vi "Get Configuration Data.vi"(8 "error in (no error)":errorcluster, 11 "Item Ref in":T18 format="%.0x") -> (0 "error out":errorcluster, 2 "framework configuration":T1, 3 "Item Ref out":T18 format="%.0x")   [LabVIEW 2017, in "DSF System Explorer.lvlib"]
uses:
  DSF System Explorer.lvlib
  <vilib>/NI Veristand/Custom Device API/Custom Device Item Ref.ctl
  DSF Core.lvlibp/Typedefs/DSF Engine Framework Configuration.ctl
  DSF Core.lvlibp/Typedefs/DSF Engine Plugin Configuration.ctl
  DSF Core.lvlibp/Typedefs/DSF Core Plugin Configuration.ctl
  DSF Core.lvlibp/Typedefs/DSF Timing Info.ctl
  DSF Core.lvlibp/Typedefs/DSF Settings Info.ctl
  DSF Core.lvlibp/Typedefs/DSF Version Info.ctl
  DSF Core.lvlibp/Typedefs/DSF Engine Plugin Thread Configuration.ctl
  DSF Core.lvlibp/Typedefs/DSF Core Thread Configuration.ctl
  DSF Core.lvlibp/Typedefs/DSF Engine Transfer Group Configuration.ctl
  DSF Core.lvlibp/Typedefs/DSF Core Group Configuration.ctl
  DSF Core.lvlibp/Typedefs/DSF Direction.ctl
  DSF Core.lvlibp/Typedefs/DSF Timeout Behavior.ctl
  DSF Core.lvlibp/Typedefs/DSF Engine Transfer Configuration.ctl
  DSF Core.lvlibp/Typedefs/DSF Core Transfer Configuration.ctl
  DSF Core.lvlibp/Typedefs/DSF Engine Channel Configuration.ctl
  DSF Core.lvlibp/Typedefs/DSF Core Channel Configuration.ctl
  DSF Core.lvlibp/Typedefs/DSF Data Type.ctl
  shared data ref.ctl
  <vilib>/NI Veristand/Custom Device API/Get Item Property (U32).vi
  <vilib>/NI Veristand/Custom Device API/Custom Device API.lvlib
  DSF Core.lvlibp
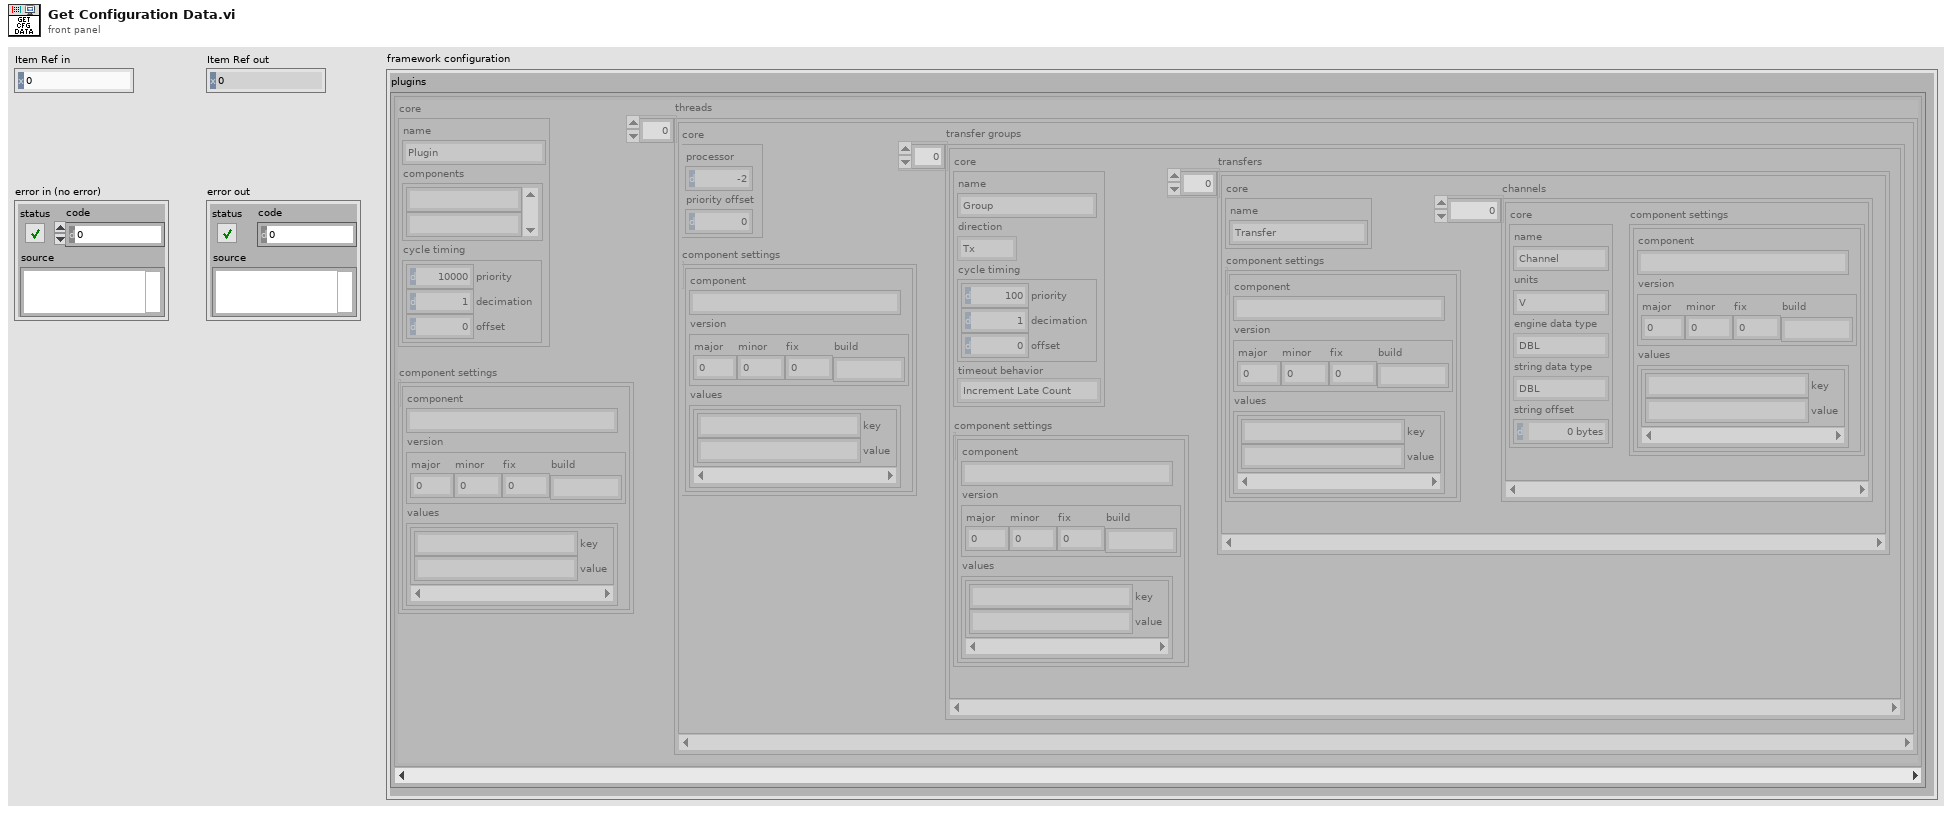
[diagram p1: front panel]
types:
  T1 = typedef "DSF Core.lvlibp/DSF Engine Framework Configuration.ctl" = cluster{"plugins":T2[]}
  T2 = typedef "DSF Core.lvlibp/DSF Engine Plugin Configuration.ctl" = cluster{"core":T3, "component settings":T5[], "threads":T7[]}
  T3 = typedef "DSF Core.lvlibp/DSF Core Plugin Configuration.ctl" = cluster{"name":string, "components":string[], "cycle timing":T4}
  T4 = typedef "DSF Core.lvlibp/DSF Timing Info.ctl" = cluster{"priority":u64, "decimation":u64, "offset":u64}
  T5 = typedef "DSF Core.lvlibp/DSF Settings Info.ctl" = cluster{"component":string, "version":T6, "values":cluster{"key":string, "value":string}[]}
  T6 = typedef "DSF Core.lvlibp/DSF Version Info.ctl" = cluster{"major":u32, "minor":u32, "fix":u32, "build":string}
  T7 = typedef "DSF Core.lvlibp/DSF Engine Plugin Thread Configuration.ctl" = cluster{"core":T8, "component settings":T5[], "transfer groups":T9[]}
  T8 = typedef "DSF Core.lvlibp/DSF Core Thread Configuration.ctl" = cluster{"processor":i32, "priority offset":i16}
  T9 = typedef "DSF Core.lvlibp/DSF Engine Transfer Group Configuration.ctl" = cluster{"core":T10, "component settings":T5[], "transfers":T13[]}
  T10 = typedef "DSF Core.lvlibp/DSF Core Group Configuration.ctl" = cluster{"name":string, "direction":T11, "cycle timing":T4, "timeout behavior":T12}
  T11 = typedef "DSF Core.lvlibp/DSF Direction.ctl" = enum8{"Tx", "Rx"}
  T12 = typedef "DSF Core.lvlibp/DSF Timeout Behavior.ctl" = enum8{"Increment Late Count", "Throw Error"}
  T13 = typedef "DSF Core.lvlibp/DSF Engine Transfer Configuration.ctl" = cluster{"core":T14, "component settings":T5[], "channels":T15[]}
  T14 = typedef "DSF Core.lvlibp/DSF Core Transfer Configuration.ctl" = cluster{"name":string}
  T15 = typedef "DSF Core.lvlibp/DSF Engine Channel Configuration.ctl" = cluster{"core":T16, "component settings":T5[]}
  T16 = typedef "DSF Core.lvlibp/DSF Core Channel Configuration.ctl" = cluster{"name":string, "units":string, "engine data type":T17, "string data type":T17, "string offset":u64}
  T17 = typedef "DSF Core.lvlibp/DSF Data Type.ctl" = enum8{"Bool", "SGL", "DBL", "I8", "I16", "I32", "I64", "U8", "U16", "U32", "U64"}
  T18 = typedef "Custom Device API.lvlib/Custom Device Item Ref.ctl" = u64
  T19 = typedef "DSF System Explorer.lvlib/shared data ref.ctl" = refnum<data-value>
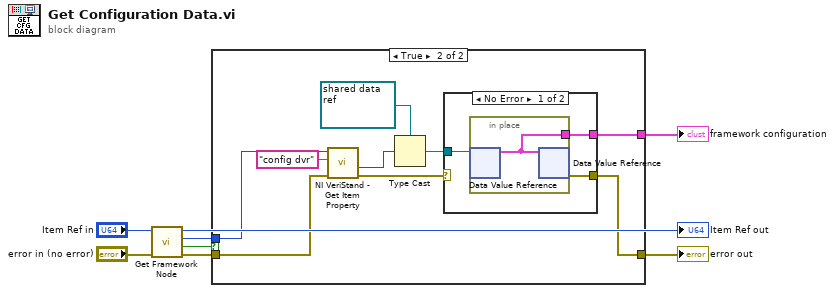
[diagram p0: block diagram]
diagram:
  n1 = call "Get Framework Node.vi"("error in (no error)"="error in (no error)", "Item Ref in"="Item Ref in") -> ("error out"=w5:errorcluster, "found?"=w2:bool, "Framework Ref"=w4:T18, "Item Ref out"=→"Item Ref out":T18)  [unwired: 6 in]
  n2 = case shown="True" w2 {
    tunnel: [_ w13] -> w8
    tunnel: w5 -> [w9 w12]
    tunnel: w4 -> [_ w11]
    tunnel: [w9 w10] -> w3
    frame False {
    }
    frame True {
      n3 = call-poly <vilib>:"NI VeriStand - Get Item Property.vi"("error in (no error)"=w12, "Property Name"="config dvr", "Item Ref in"=w11) -> ("error out"=w14:errorcluster, "Value"=w16:u32)  [unwired: 5 in, 2 out]
      n4 = Type Cast(type=T19 refnum ("data value reference"), x=w16) -> (*(type *) &x=w15:T19)
      n5 = case shown="No Error" w14 {
        selector: w14 -> [_ w23]
        tunnel: w15 -> [w21 _]
        tunnel: [w20 w23] -> w10
        tunnel: [w19 _] -> w13
        frame No Error {
          n6 = in-place {
            in-place-border: [w22] -> w19
            n7 = in-place-dvr #1(w21) -> (w22:T1)  [unwired: 1 out]
            n8 = in-place-dvr #1(w22) -> (w20:errorcluster)  [unwired: 1 out]
          }
        }
        frame Error {
        }
      }
    }
  }
  "error out" <- w3
  "framework configuration" <- w8
